vi "GetSetPowerFailRecovery.vi"(0 "VISA resource name":refnum<visa-resource-name>, 1 "get/set":T3, 2 "Enabled?":T2 items=["Off", "On"], 3 "Time":u16 max=300 step=1, 4 "Power Recovery Mode":T1 items=["stop", "hold", "run", "restart"], 5 "error in":errorcluster) -> (14 "VISA resource name out":refnum<visa-resource-name>, 15 "Power fail recovery response":string, 19 "error out":errorcluster)   [LabVIEW 2023, in "Thermotron 8800.lvlib"]
doc: "PWRF\nCommand name: Send or load power fail recovery settings.\nCommand type: Variable\nDescription: This command is for setting the power failure recovery options. For more information, refer to “Power failure recovery” in Section 1 of this manual. The query command asks the 8800 for the current power fail recovery settings. The operation command allows you to modify the settings.\nSyntax: PWRF? or PWRFenabled, time, mode\nWhere:\nenabled = 1 = on; 0 = off\ntime = maximum off time in minutes from 0 to 300 (5 hours)\nmode = 0 = stop; 1 = hold; 2 = run; 3 = restart\nQuery example: PWRF?\n8800 response: 1, 45, 0 (Power fail recovery is enabled, the maximum off time is 45 minutes, and the recovery mode is stop.)\nOperation example 1: PWRF1, 15, 3\n8800 response: 0 (The 8800 will enable power fail recovery, set the maximum off time to 15 minutes, and set the recovery mode to restart.)\nOperation example 2: PWRF0\n8800 response: 0 (The 8800 will disable power fail recovery.)"
uses:
  Thermotron 8800.lvlib
  Private/get set.ctl
  Private/Enabled Off On.ctl
  Private/Power Recovery Mode.ctl
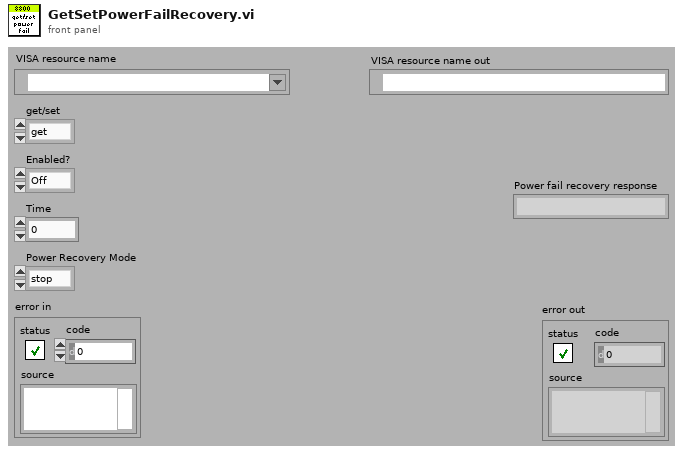
[diagram p1: front panel]
types:
  T1 = typedef "Thermotron 8800.lvlib/Power Recovery Mode.ctl" = u8
  T2 = typedef "Thermotron 8800.lvlib/Enabled Off On.ctl" = u8
  T3 = typedef "Thermotron 8800.lvlib/get set.ctl" = enum16{"get", "set"}
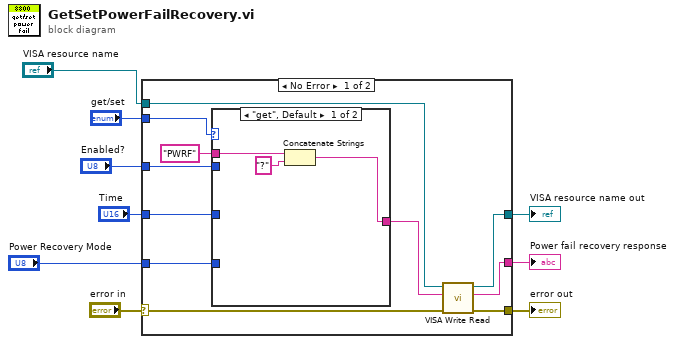
[diagram p0: block diagram]
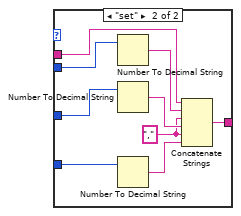
[diagram p2: hidden frame]
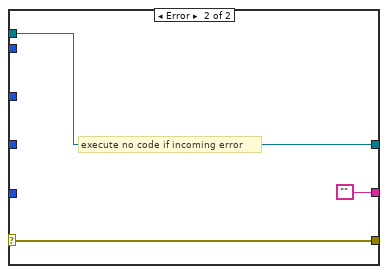
[diagram p3: hidden frame]
diagram:
  n1 = case shown="No Error" "error in" {
    selector: "error in" -> [w13 w34]
    tunnel: "get/set" -> [w20 _]
    tunnel: [w18 ""] -> w3
    tunnel: [w17 w34] -> w7
    tunnel: [w16 w35] -> w6
    tunnel: "VISA resource name" -> [w15 w35]
    tunnel: "Time" -> [w14 _]
    tunnel: "Enabled?" -> [w12 _]
    tunnel: "Power Recovery Mode" -> [w11 _]
    frame No Error {
      n2 = case shown="\"get\", Default" w20 {
        tunnel: "PWRF" ("8800 Command") -> [w22 w32]
        tunnel: [w23 w31] -> w10
        tunnel: w14 -> [_ w30]
        tunnel: w12 -> [_ w29]
        tunnel: w11 -> [_ w28]
        frame "get", Default {
          n3 = Concatenate Strings(w22, "?" ("8800 Command")) -> (w23:string)
        }
        frame "set" {
          w25 = ","
          n4 = Number To Decimal String(number=w29) -> (decimal integer string=w27:string)  [unwired: 1 in]
          n5 = Number To Decimal String(number=w30) -> (decimal integer string=w26:string)  [unwired: 1 in]
          n6 = Number To Decimal String(number=w28) -> (decimal integer string=w24:string)  [unwired: 1 in]
          n7 = Concatenate Strings(w32, w27, w25, w26, w25, w24) -> (w31:string)
        }
      }
      n8 = call "VISA Write Read.vi"("error in (no error)"=w13, "8800 Command"=w10, "VISA Refnum in"=w15) -> ("error out"=w17:errorcluster, "read buffer"=w18:string, "VISA Refnum out"=w16:refnum<visa-resource-name>)  [unwired: 6 in]
    }
    frame Error {
      # "execute no code if incoming error"
    }
  }
  "VISA resource name out" <- w6
  "error out" <- w7
  "Power fail recovery response" <- w3
